vi "Create Group Transfers.vi"(7 "direction":T2, 8 "error in (no error)":errorcluster, 9 "Group ID":string, 10 "dsf refnum in":refnum<class "Configuration Session.lvclass">, 11 "Section Ptr":T1 format="%.0x") -> (0 "error out":errorcluster)   [LabVIEW 2017, in "DSF System Explorer.lvlib"]
uses:
  DSF System Explorer.lvlib
  DSF Core.lvlibp/Typedefs/DSF Direction.ctl
  DSF Core.lvlibp/Classes/Configuration/Configuration Session.lvclass
  <vilib>/NI Veristand/Custom Device API/Custom Device Item Ref.ctl
  DSF Core.lvlibp/Classes/Configuration/Read Group Transfer IDs.vi
  Shared/Transfer Page GUID.vi
  <vilib>/NI Veristand/Custom Device API/Set Item Property (String).vi
  <vilib>/NI Veristand/Custom Device API/Custom Device API.lvlib
  Shared/DSF Shared.lvlib
  DSF Core.lvlibp
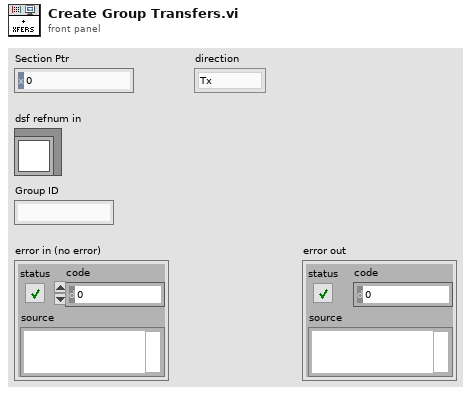
[diagram p1: front panel]
types:
  T1 = typedef "Custom Device API.lvlib/Custom Device Item Ref.ctl" = u64
  T2 = typedef "DSF Core.lvlibp/DSF Direction.ctl" = enum8{"Tx", "Rx"}
  T3 = typedef "DSF System Explorer.lvlib/shared data ref.ctl" = refnum<data-value>
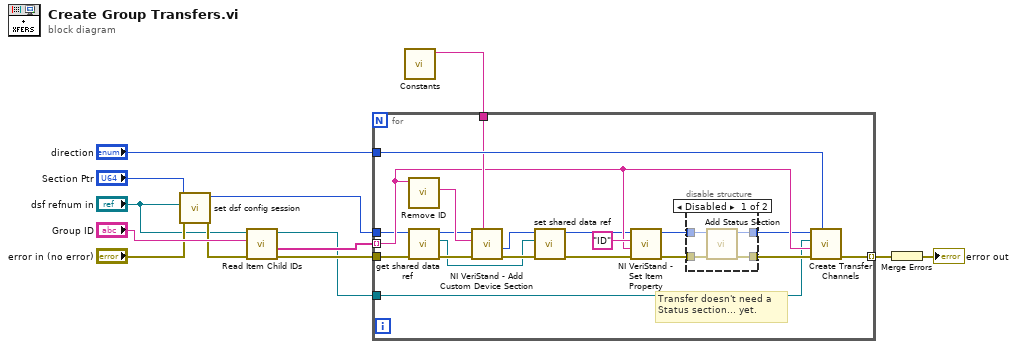
[diagram p0: block diagram]
diagram:
  n1 = call "set dsf config session.vi"("error in (no error)"="error in (no error)", "Configuration Session"="dsf refnum in", "Item Ref in"="Section Ptr") -> ("error out"=w5:errorcluster, "Item Ref out"=w1:T1)  [unwired: 7 in]
  n2 = call-poly "Read Item Child IDs.vi"("error in (no error)"=w5, "Group ID"="Group ID", "Configuration Session in"="dsf refnum in") -> ("error out"=w9:errorcluster, "Transfer IDs"=w8:string[], "Configuration Session out"=w3:refnum<class "Configuration Session.lvclass">)  [unwired: 5 in, 1 out]
  n3 = call-poly "Constants.vi"() -> ("Transfer GUID"=w2:string)  [unwired: 11 in]
  n4 = for {
    tunnel: w8 -> [w28] mode=indexing
    tunnel: w9 -> [w26]
    tunnel: [w33] -> w12 mode=indexing
    tunnel: w1 -> [w27]
    tunnel: w3 -> [w14]
    tunnel: "direction" -> [w32]
    tunnel: w2 -> [w30]
    # "Transfer doesn't need a Status section... yet."
    n5 = call "Remove ID.vi"("id string"=w28) -> ("name"=w31:string)  [unwired: 8 in, 2 out]
    n6 = call "get shared data ref.vi"("error in (no error)"=w26, "Item Ref in"=w27) -> ("error out"=w24:errorcluster, "shared data ref"=w21:T3, "Item Ref out"=w25:T1)  [unwired: 7 in]
    n7 = call <vilib>:"NI VeriStand - Add Custom Device Section.vi"("GUID (Default Section)"=w30, "error in (no error)"=w24, "Section Name"=w31, "Parent Ref in"=w25) -> ("error out"=w23:errorcluster, "Section Ptr"=w22:T1)  [unwired: 4 in, 2 out]
    n8 = call "set shared data ref.vi"("error in (no error)"=w23, "shared data ref"=w21, "Node Ptr"=w22) -> ("error out"=w19:errorcluster, "Item Ref out"=w20:T1)  [unwired: 7 in]
    n9 = call-poly <vilib>:"NI VeriStand - Set Item Property.vi"("error in (no error)"=w19, "Value"=w28, "Property Name"="ID", "Item Ref in"=w20) -> ("error out"=w17:errorcluster, "Item Ref out"=w18:T1)  [unwired: 5 in, 1 out]
    n10 = disable-structure shown="Disabled" {
      disable-tunnel: w18 -> [w37 w39]
      disable-tunnel: w17 -> [w36 w38]
      disable-tunnel: [w35 w38] -> w16
      disable-tunnel: [w34 w39] -> w15
      frame Disabled {
        n11 = call "Add Status Section.vi"("error in (no error)"=w36, "Item Ref in"=w37) -> ("error out"=w35:errorcluster, "Item Ref out"=w34:T1)  [unwired: 8 in]
      }
      frame Enabled {
      }
    }
    n12 = call "Create Transfer Channels.vi"("direction"=w32, "error in (no error)"=w16, "Transfer ID"=w28, "Refnum in"=w14, "Section Ptr"=w15) -> ("error out"=w33:errorcluster)  [unwired: 6 in]
  }
  n13 = Merge Errors(w12) -> (→"error out":errorcluster)
